vi "iWorx Pulse SubVI.vi"(7 "Pulse Chart":refnum<vi>, 10 "Threshold (.5mV)":dbl=0.0005) -> (1 "Pulse Times":timestamp[](array[timestamp]), 2 "Inst Pulse Rate (BPM)":dbl, 3 "Average Pulse Rate (BPM)":dbl)   [LabVIEW 2012]
doc: "This subVI uses a Reference from a Waveform Chart in order to extract the data visible on the chart. It then calculates when pulse beats occur based on a simple negative threshold. This function returns the <b>Instantaneous Pulse</b> based on your last two heart beats as well as the <b>Average Pulse</b> from the data visible on the chart."
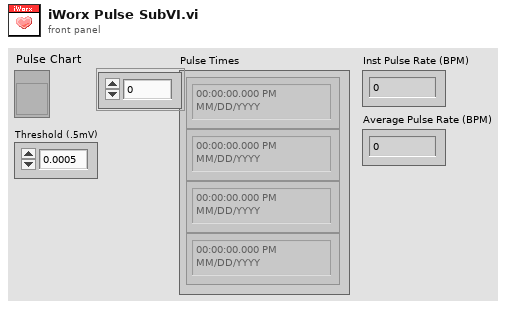
[diagram p1: front panel]
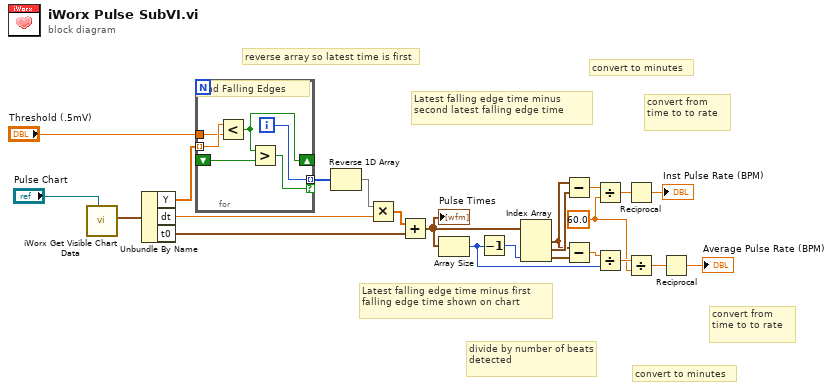
[diagram p0: block diagram]
diagram:
  w8 = 60.0 ("y")
  # "reverse array so latest time is first"
  # "convert to minutes"
  # "divide by number of beats detected"
  # "convert from time to to rate"
  # "convert from time to to rate"
  # "convert to minutes"
  # "Latest falling edge time minus first falling edge time shown on chart"
  # "Latest falling edge time minus second latest falling edge time"
  n1 = call "iWorx Get Visible Chart Data.vi"("Selection Chart"="Pulse Chart") -> ("waveform out"=w23:waveform(dbl))  [unwired: 8 in, 2 out]
  n2 = Unbundle By Name(w23) -> ("Y"=w22:dbl[], "dt"=w21:dbl, "t0"=w19:timestamp)
  n3 = for {
    tunnel: w22 -> [w29] mode=indexing
    tunnel: "Threshold (.5mV)" -> [w28]
    shift-right: [w27] -> _
    shift-left: _ -> [w26]
    tunnel: [w25] -> w18 mode=indexing if=w24
    i -> [w25]
    # "Find Falling Edges"
    n4 = Less?(x=w29, y=w28) -> (x < y?=w27:bool)
    n5 = Greater?(x=w27, y=w26) -> (0:w24:bool)
  }
  n6 = Reverse 1D Array(array=w18) -> (reversed array=w17:i32[])
  n7 = Multiply(x=w17, y=w21) -> (x*y=w20:dbl[])
  n8 = Add(x=w20, y=w19) -> (x+y=w5:timestamp[])
  "Pulse Times" <- w5
  n9 = Array Size(array=w5) -> (size(s)=w10:i32)
  n10 = Decrement(x=w10) -> (x-1=w16:i32)
  n11 = Index Array(array=w5, index #3=w16) -> (element #1=w14:timestamp, element #2=w15:timestamp, element #3=w13:timestamp)  [unwired: 2 in]
  n12 = Subtract(x=w14, y=w15) -> (x-y=w12:dbl)
  n13 = Subtract(x=w14, y=w13) -> (x-y=w11:dbl)
  n14 = Divide(x=w12, y=w8) -> (x/y=w7:dbl)
  n15 = Divide(x=w11, y=w10) -> (x/y=w9:dbl)
  n16 = Reciprocal(x=w7) -> (1/x=→"Inst Pulse Rate (BPM)":dbl)
  n17 = Divide(x=w9, y=w8) -> (x/y=w6:dbl)
  n18 = Reciprocal(x=w6) -> (1/x=→"Average Pulse Rate (BPM)":dbl)
